vi "T7MOD_Write_INT32_Register.vi"(7 "INT32 to Write":i32=-123, 8 "error in":errorcluster, 9 "LabJack INT32 Register":i32=55122, 10 "Remote Port":u16=502, 11 "Remote IP Address":string="192.168.1.15") -> (0 "error out":errorcluster, 1 "Written At":timestamp)   [LabVIEW 2018]
panel:
  # "Input"
  # "TCP Parameters"
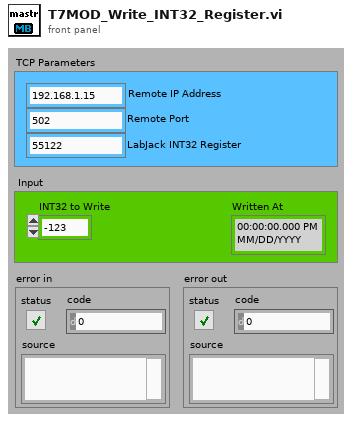
[diagram p1: front panel]
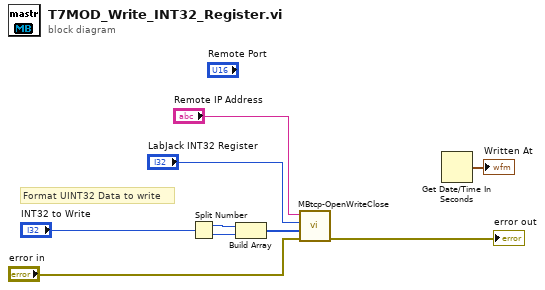
[diagram p0: block diagram]
diagram:
  # "Format UINT32 Data to write"
  n1 = Split Number(x="INT32 to Write") -> (hi(x)=w8:u16, lo(x)=w7:u16)
  n2 = Build Array(w8, w7) -> (w3:u16[])
  n3 = call "MBtcp-OpenWriteClose.vi"("error in (no error)"="error in", "Values"=w3, "RegisterAddr"="LabJack INT32 Register", "IP Address(:port)"="Remote IP Address") -> ("error out"=→"error out":errorcluster)  [unwired: 7 in]
  n4 = Get Date/Time In Seconds() -> (seconds since 1Jan1904=→"Written At":timestamp)
